vi "Configure Pulse Waveform.vi"(5 "Trailing Edge Time (7.5E-9 Seconds)":dbl=7.5e-09, 6 "Delay (0.0 Seconds)":dbl, 7 "Leading Edge Time (7.5E-9 Seconds)":dbl=7.5e-09, 8 "error in (no error)":errorcluster, 9 "Duty Cycle (50.0 %)":dbl=50.0, 10 "Channel (1: Channel1)":u16(ring)=1 items=["Channel1"=1, "Channel2"=2], 11 "VISA resource name":refnum<visa-resource-name>) -> (0 "error out":errorcluster, 3 "VISA resource name out":refnum<visa-resource-name>)   [LabVIEW 2009, in "Agilent 81150.lvlib"]
doc: "Configures parameters for pulse waveforms which include channel, leading edge time, trailing edge time, duty cycle, and delay."
uses:
  Agilent 81150.lvlib
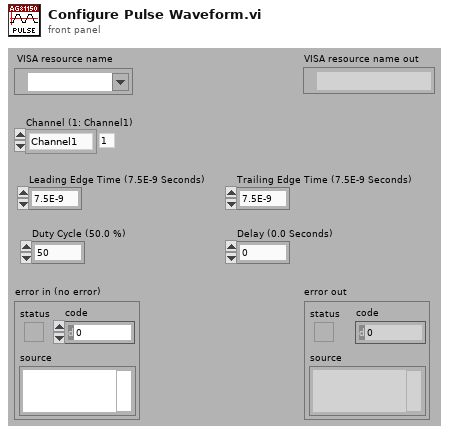
[diagram p1: front panel]
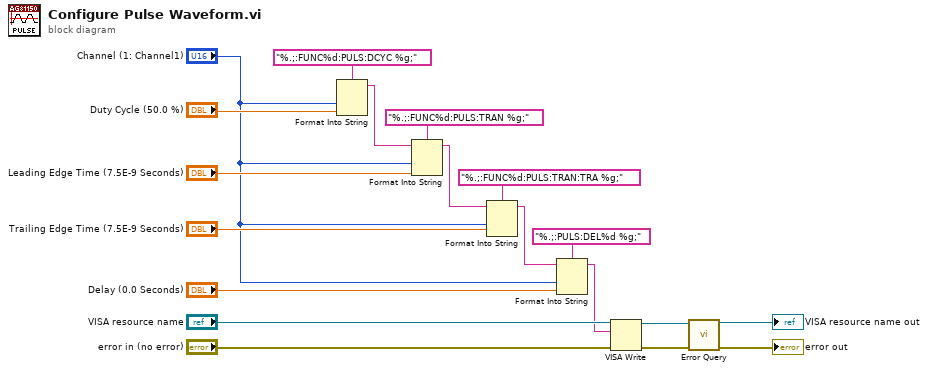
[diagram p0: block diagram]
diagram:
  n1 = Format Into String(format string="%.;:FUNC%d:PULS:DCYC %g;", "Channel (1: Channel1)", "Duty Cycle (50.0 %)") -> (resulting string=w16:string)  [unwired: 2 in, 1 out]
  n2 = Format Into String(format string="%.;:FUNC%d:PULS:TRAN %g;", initial string=w16, "Channel (1: Channel1)", "Leading Edge Time (7.5E-9 Seconds)") -> (resulting string=w13:string)  [unwired: 1 in, 1 out]
  n3 = Format Into String(format string="%.;:FUNC%d:PULS:TRAN:TRA %g;", initial string=w13, "Channel (1: Channel1)", "Trailing Edge Time (7.5E-9 Seconds)") -> (resulting string=w2:string)  [unwired: 1 in, 1 out]
  n4 = Format Into String(format string="%.;:PULS:DEL%d %g;", initial string=w2, "Channel (1: Channel1)", "Delay (0.0 Seconds)") -> (resulting string=w1:string)  [unwired: 1 in, 1 out]
  n5 = VISA Write(VISA resource name="VISA resource name", write buffer=w1, error in (no error)="error in (no error)") -> (VISA resource name out=w9:refnum<visa-resource-name>, error out=w8:errorcluster)  [unwired: 1 out]
  n6 = call "Error Query.vi"("error in (no error)"=w8, "VISA resource name"=w9) -> ("error out"=→"error out":errorcluster, "VISA resource name out"=→"VISA resource name out":refnum<visa-resource-name>)  [unwired: 8 out]
